vi "MFR Flow to SP 2-2_RS232.vi"(6 "Omicron":bool, 8 "MFC Size":dbl[](array[numeric]), 10 "MFC SPs":dbl[](array[numeric])) -> (2 "MFC array":u8[](array[numeric]), 4 "SV Array":bool[](array[boolean]))   [LabVIEW 2014]
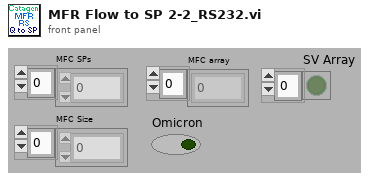
[diagram p1: front panel]
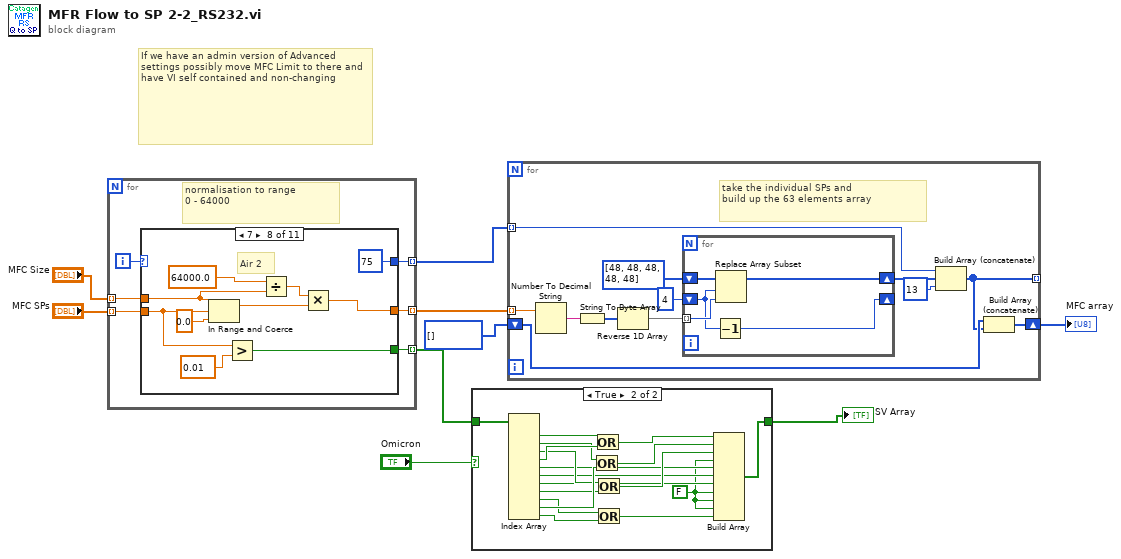
[diagram p0: block diagram]
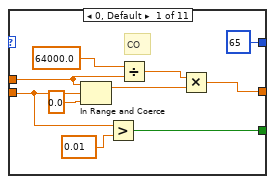
[diagram p3: hidden frame]
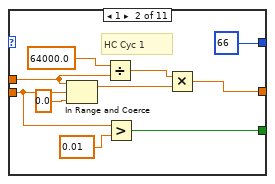
[diagram p4: hidden frame]
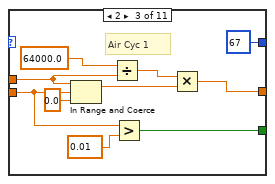
[diagram p5: hidden frame]
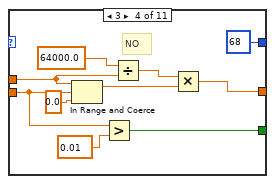
[diagram p6: hidden frame]
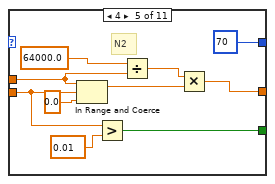
[diagram p7: hidden frame]
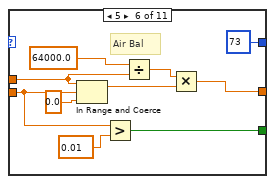
[diagram p8: hidden frame]
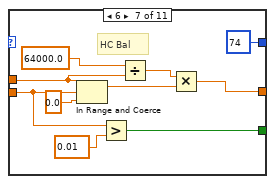
[diagram p9: hidden frame]
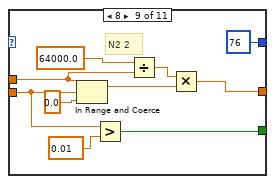
[diagram p10: hidden frame]
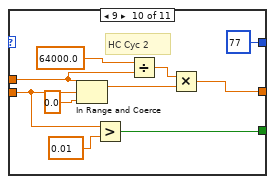
[diagram p11: hidden frame]
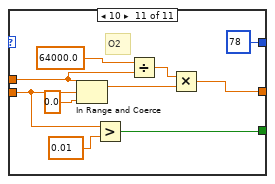
[diagram p12: hidden frame]
diagram:
  # "If we have an admin version of Advanced settings possibly move MFC Limit to there and have VI self contained and non-changing"
  n1 = for {
    tunnel: "MFC SPs" -> [w14] mode=indexing
    tunnel: [w13] -> w6 mode=indexing
    tunnel: [w12] -> w5 mode=indexing
    tunnel: [w11] -> w3 mode=indexing
    tunnel: "MFC Size" -> [w10] mode=indexing
    i -> [w15]
    # "normalisation to range\n0 - 64000"
    n2 = case shown="7" w15 {
      tunnel: w14 -> [w17 w27 w37 w47 w57 w67 w77 w89 w99 w109 w119]
      tunnel: [w21 w35 w45 w50 w65 w75 w85 w95 w105 w115 w125] -> w13
      tunnel: [u8 65 ("y") u8 66 ("y") u8 67 ("y") u8 68 ("y") u8 70 ("y") u8 73 ("y") u8 74 ("y") u8 75 ("y") u8 76 ("y") u8 77 ("y") u8 78 ("y")] -> w12
      tunnel: [w18 w28 w38 w48 w58 w68 w78 w87 w97 w107 w117] -> w11
      tunnel: w10 -> [w16 w26 w36 w46 w56 w66 w76 w86 w96 w106 w116]
      frame 0, Default {
        # "CO"
        n3 = In Range and Coerce(upper limit=w16, x=w17, lower limit=0.0) -> (coerced(x)=w23:dbl)  [unwired: 1 out]
        n4 = Greater?(x=w17, y=0.01) -> (0:w18:bool)
        n5 = Divide(x=64000.0, y=w16) -> (x/y=w22:dbl)
        n6 = Multiply(x=w22, y=w23) -> (x*y=w21:dbl)
      }
      frame 1 {
        # "HC Cyc 1"
        n7 = In Range and Coerce(upper limit=w26, x=w27, lower limit=0.0) -> (coerced(x)=w32:dbl)  [unwired: 1 out]
        n8 = Divide(x=64000.0, y=w26) -> (x/y=w30:dbl)
        n9 = Greater?(x=w27, y=0.01) -> (0:w28:bool)
        n10 = Multiply(x=w30, y=w32) -> (x*y=w35:dbl)
      }
      frame 2 {
        # "Air Cyc 1"
        n11 = In Range and Coerce(upper limit=w36, x=w37, lower limit=0.0) -> (coerced(x)=w42:dbl)  [unwired: 1 out]
        n12 = Divide(x=64000.0, y=w36) -> (x/y=w41:dbl)
        n13 = Greater?(x=w37, y=0.01) -> (0:w38:bool)
        n14 = Multiply(x=w41, y=w42) -> (x*y=w45:dbl)
      }
      frame 3 {
        # "NO"
        n15 = In Range and Coerce(upper limit=w46, x=w47, lower limit=0.0) -> (coerced(x)=w53:dbl)  [unwired: 1 out]
        n16 = Greater?(x=w47, y=0.01) -> (0:w48:bool)
        n17 = Divide(x=64000.0, y=w46) -> (x/y=w52:dbl)
        n18 = Multiply(x=w52, y=w53) -> (x*y=w50:dbl)
      }
      frame 4 {
        # "N2"
        n19 = In Range and Coerce(upper limit=w56, x=w57, lower limit=0.0) -> (coerced(x)=w61:dbl)  [unwired: 1 out]
        n20 = Greater?(x=w57, y=0.01) -> (0:w58:bool)
        n21 = Divide(x=64000.0, y=w56) -> (x/y=w60:dbl)
        n22 = Multiply(x=w60, y=w61) -> (x*y=w65:dbl)
      }
      frame 5 {
        # "Air Bal"
        n23 = In Range and Coerce(upper limit=w66, x=w67, lower limit=0.0) -> (coerced(x)=w72:dbl)  [unwired: 1 out]
        n24 = Greater?(x=w67, y=0.01) -> (0:w68:bool)
        n25 = Divide(x=64000.0, y=w66) -> (x/y=w70:dbl)
        n26 = Multiply(x=w70, y=w72) -> (x*y=w75:dbl)
      }
      frame 6 {
        # "HC Bal"
        n27 = In Range and Coerce(upper limit=w76, x=w77, lower limit=0.0) -> (coerced(x)=w82:dbl)  [unwired: 1 out]
        n28 = Greater?(x=w77, y=0.01) -> (0:w78:bool)
        n29 = Divide(x=64000.0, y=w76) -> (x/y=w80:dbl)
        n30 = Multiply(x=w80, y=w82) -> (x*y=w85:dbl)
      }
      frame 7 {
        # "Air 2"
        n31 = In Range and Coerce(upper limit=w86, x=w89, lower limit=0.0) -> (coerced(x)=w92:dbl)  [unwired: 1 out]
        n32 = Greater?(x=w89, y=0.01) -> (0:w87:bool)
        n33 = Divide(x=64000.0, y=w86) -> (x/y=w90:dbl)
        n34 = Multiply(x=w90, y=w92) -> (x*y=w95:dbl)
      }
      frame 8 {
        # "N2 2"
        n35 = In Range and Coerce(upper limit=w96, x=w99, lower limit=0.0) -> (coerced(x)=w102:dbl)  [unwired: 1 out]
        n36 = Greater?(x=w99, y=0.01) -> (0:w97:bool)
        n37 = Divide(x=64000.0, y=w96) -> (x/y=w100:dbl)
        n38 = Multiply(x=w100, y=w102) -> (x*y=w105:dbl)
      }
      frame 9 {
        # "HC Cyc 2"
        n39 = In Range and Coerce(upper limit=w106, x=w109, lower limit=0.0) -> (coerced(x)=w112:dbl)  [unwired: 1 out]
        n40 = Greater?(x=w109, y=0.01) -> (0:w107:bool)
        n41 = Divide(x=64000.0, y=w106) -> (x/y=w110:dbl)
        n42 = Multiply(x=w110, y=w112) -> (x*y=w115:dbl)
      }
      frame 10 {
        # "O2"
        n43 = In Range and Coerce(upper limit=w116, x=w119, lower limit=0.0) -> (coerced(x)=w122:dbl)  [unwired: 1 out]
        n44 = Greater?(x=w119, y=0.01) -> (0:w117:bool)
        n45 = Divide(x=64000.0, y=w116) -> (x/y=w120:dbl)
        n46 = Multiply(x=w120, y=w122) -> (x*y=w125:dbl)
      }
    }
  }
  n47 = case shown="True" "Omicron" {
    tunnel: w3 -> [w126 w144]
    tunnel: [w126 w127] -> w2
    frame False {
      # "Omega"
    }
    frame True {
      w128 = FALSE ("element")
      n48 = Index Array(array=w144) -> (element #1=w143:bool, element #2=w140:bool, element #3=w135:bool, element #4=w142:bool, element #5=w131:bool, element #6=w130:bool, element #7=w129:bool, element #8=w136:bool, element #9=w132:bool, element #10=w139:bool, element #11=w133:bool)  [unwired: 11 in]
      n49 = Or(x=w140, y=w139) -> (x .or. y?=w138:bool)
      n50 = Or(x=w143, y=w142) -> (x .or. y?=w141:bool)
      n51 = Or(x=w135, y=w136) -> (x .or. y?=w137:bool)
      n52 = Or(x=w132, y=w133) -> (x .or. y?=w134:bool)
      n53 = Build Array(w141, w138, w137, w128, w131, w130, w129, w128, w128, w128, w134) -> (w127:bool[])
    }
  }
  "SV Array" <- w2
  n54 = for {
    tunnel: w5 -> [w151] mode=indexing
    tunnel: [w147] -> _ mode=indexing
    shift-right: [w146] -> w8
    shift-left: u8[] [] -> [w148]
    tunnel: w6 -> [w145] mode=indexing
    # "take the individual SPs and \nbuild up the 63 elements array"
    n55 = Number To Decimal String(number=w145) -> (decimal integer string=w152:string)  [unwired: 1 in]
    n56 = String To Byte Array(string=w152) -> (unsigned byte array=w155:u8[])
    n57 = Reverse 1D Array(array=w155) -> (reversed array=w156:u8[])
    n58 = for {
      tunnel: w156 -> [w159] mode=indexing
      shift-right: [w158] -> _
      shift-left: u8 4 -> [w157]
      shift-right: [w160] -> w149
      shift-left: u8[] [48, 48, 48, 48, 48] -> [w161]
      n59 = Decrement(x=w157) -> (x-1=w158:u8)
      n60 = Replace Array Subset(array=w161, new element=w159, index=w157) -> (w160:u8[])
    }
    n61 = Build Array (concatenate)(w151, w149, u8 13) -> (w147:u8[])
    n62 = Build Array (concatenate)(w148, w147) -> (w146:u8[])
  }
  "MFC array" <- w8
